vi "Test Decimation.vi"() -> ()   [LabVIEW 2019]
uses:
  <vilib>/Analysis/baseanly.llb/Mean (DBL).vi
  <vilib>/Utility/error.llb/Clear Errors.vi
  <vilib>/Analysis/2dsp.llb/Decimate (single shot).vi
  <vilib>/Analysis/2dsp.llb/Decimate (single shot, DBL).vi
  src/DSP/Factorize Integer.vi
  <vilib>/measure/NI_MABase.lvlib
  src/DSP/DSP.lvclass
  <vilib>/Analysis/NI_AALBase.lvlib
panel:
  out "Decimation Factor":i32
  out "Waveform Graph":waveform(dbl)[](graph)
  out "XY Graph 2":cluster{i32[], dbl[]}[](graph)
  out "elapsed":dbl
  out "Method (0/1/2)":i32
  out "Decimating":i32
  out "Fs":dbl
  out "XY Graph":cluster{"Fs":dbl[], dbl[]}[](graph)
  out "Average Time\n(Decimate, Multistage, Array)":dbl[](array[numeric]) format="%#_6p"
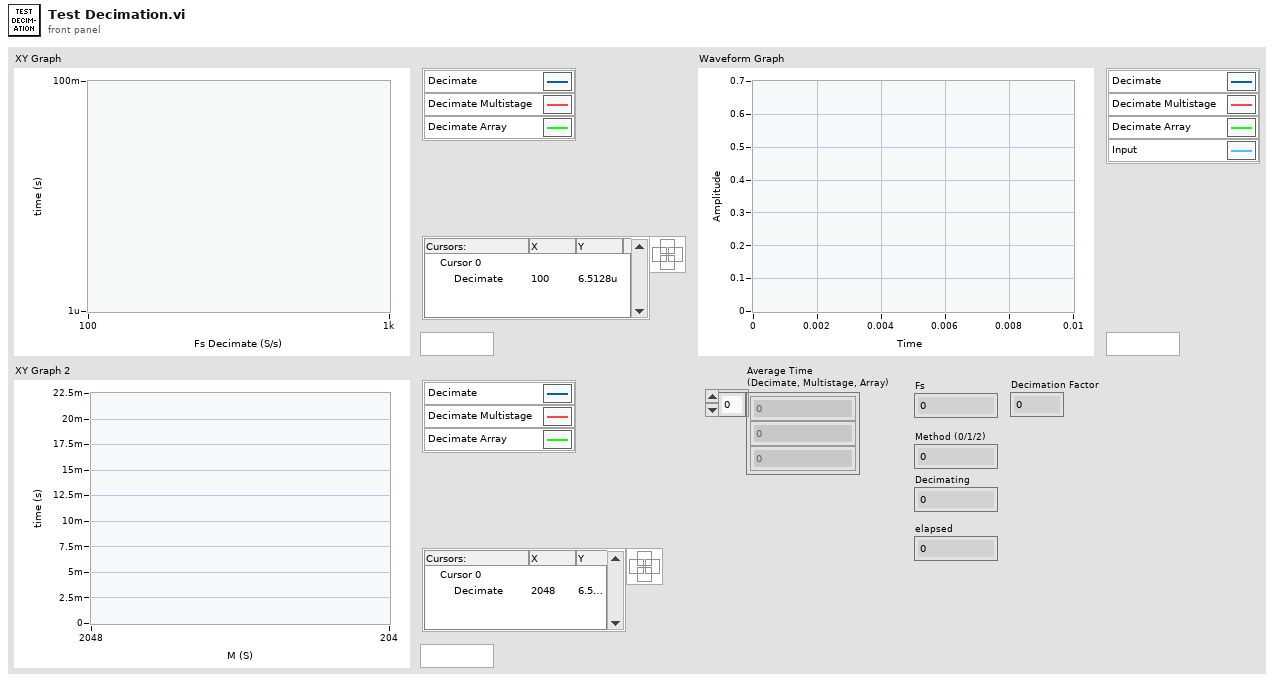
[diagram p1: front panel]
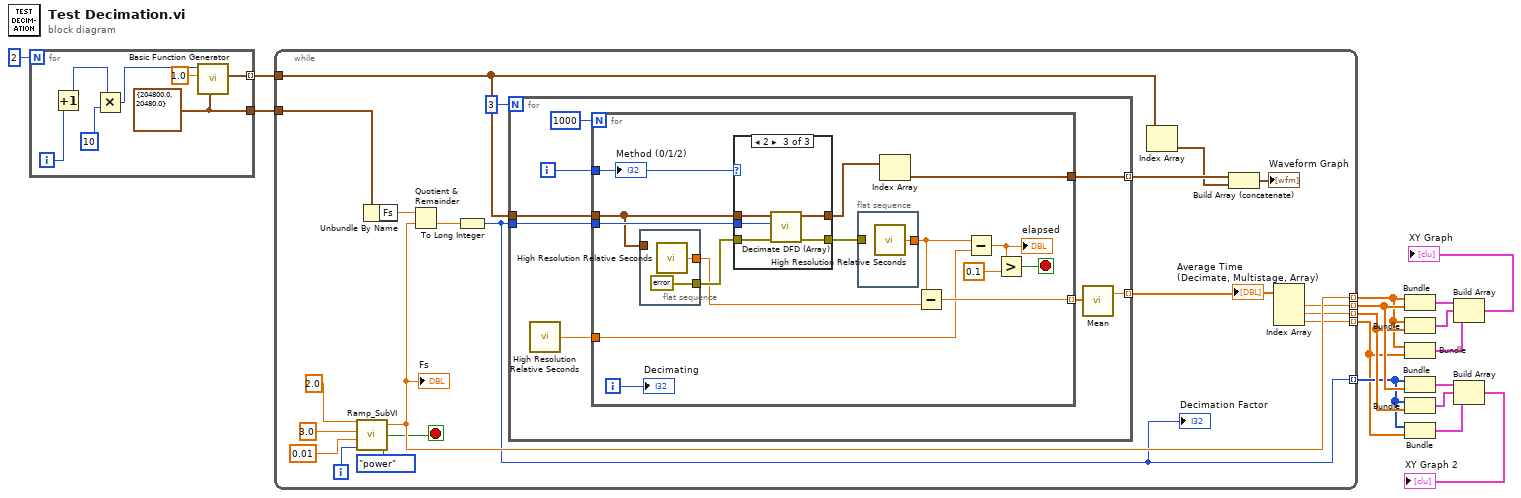
[diagram p0: block diagram]
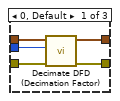
[diagram p2: hidden frame]
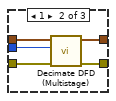
[diagram p3: hidden frame]
diagram:
  n1 = for {
    N: 2 -> [_]
    tunnel: [w23] -> w1 mode=indexing
    tunnel: [w21] -> w15
    i -> [w22]
    w21 = cluster{"Fs":dbl, "#s":dbl} {"Fs"=204800.0, "#s"=20480.0} ("sampling info")
    n2 = Increment(x=w22) -> (x+1=w18:i32)
    n3 = Multiply(x=w18, y=10) -> (x*y=w17:i32)
    n4 = call <vilib>:"Basic Function Generator.vi"("sampling info"=w21, "amplitude"=1.0, "frequency"=w17) -> ("signal out"=w23:waveform(dbl))  [unwired: 6 in, 2 out]
  }
  n5 = while {
    tunnel: w1 -> [w24]
    tunnel: w15 -> [w25]
    tunnel: [w40] -> w5 mode=indexing
    tunnel: [w34] -> w11 mode=indexing
    tunnel: [w26] -> w6 mode=indexing
    tunnel: [w33] -> w10 mode=indexing
    tunnel: [w31] -> w4 mode=indexing
    i -> [w39]
    stop <- w27 stop-if-true
    n6 = call <userlib>:"Ramp_SubVI.vi"("Enum"=enum16{"linear", "power"}."power", "index"=w39, "step"=0.01, "end"=3.0, "start"=2.0) -> ("Stop?"=w27:bool, "Numeric"=w40:dbl)
    "Fs" <- w40
    n7 = Unbundle By Name(w25) -> ("Fs"=w42:dbl)
    n8 = Quotient & Remainder(x=w42, y=w40) -> (floor(x/y)=w32:dbl)  [unwired: 1 out]
    n9 = To Long Integer(number=w32) -> (32bit integer=w26:i32)
    "Decimation Factor" <- w26
    n10 = for {
      N: 3 -> [_]
      tunnel: w24 -> [w48]
      tunnel: [w46] -> w41 mode=indexing
      tunnel: w26 -> [w49]
      tunnel: [w44] -> w29 mode=indexing
      i -> [w50]
      n11 = call <vilib>:"High Resolution Relative Seconds.vi"() -> ("relative seconds"=w45:dbl)
      n12 = for {
        N: 1000 -> [_]
        tunnel: w50 -> [w66]
        tunnel: w49 -> [w65]
        tunnel: w48 -> [w52]
        tunnel: [w57] -> w47 mode=indexing
        tunnel: w45 -> [w55]
        tunnel: [w53] -> w44
        i -> [w61]
        stop <- w63 stop-if-true
        n13 = flat-sequence {
          tunnel: [w68] -> w58
          tunnel: w52 -> [_]
          tunnel: [errorcluster {"status"=FALSE, "code"=0, "source"=""} ("error in (no error)")] -> w59
          frame #0 {
            n14 = call <vilib>:"High Resolution Relative Seconds.vi"() -> ("relative seconds"=w68:dbl)
          }
        }
        n15 = case shown="2" w66 {
          tunnel: w52 -> [w74 w79 w84]
          tunnel: [w73 w78 w81] -> w60
          tunnel: w65 -> [w72 w77 w82]
          tunnel: w59 -> [w71 w76 w83]
          tunnel: [w70 w75 w80] -> w54
          frame 0, Default {
            n16 = call "Decimate DFD (Decimation Factor).vi"("error in (no error)"=w71, "Decimation Factor"=w72, "Waveforms in"=w74) -> ("error out"=w73:errorcluster, "waveforms out"=w70:waveform(dbl)[])  [unwired: 7 in]
          }
          frame 1 {
            n17 = call "Decimate DFD (Multistage).vi"("error in (no error)"=w76, "Decimation Factor"=w77, "Waveforms in"=w79) -> ("error out"=w78:errorcluster, "waveforms out"=w75:waveform(dbl)[])  [unwired: 7 in]
          }
          frame 2 {
            n18 = call "Decimate DFD (Array).vi"("error in (no error)"=w83, "Decimation Factor"=w82, "Waveforms in"=w84) -> ("error out"=w81:errorcluster, "waveforms out"=w80:waveform(dbl)[])  [unwired: 7 in]
          }
        }
        n19 = flat-sequence {
          tunnel: [w69] -> w56
          tunnel: w60 -> [_]
          frame #0 {
            n20 = call <vilib>:"High Resolution Relative Seconds.vi"() -> ("relative seconds"=w69:dbl)
          }
        }
        n21 = Index Array(array=w54) -> (element=w53:waveform(dbl))  [unwired: 1 in]
        n22 = Subtract(x=w56, y=w58) -> (x-y=w57:dbl)
        n23 = Subtract(x=w56, y=w55) -> (x-y=w64:dbl)
        "elapsed" <- w64
        n24 = Greater?(x=w64, y=0.1) -> (0:w63:bool)
        "Decimating" <- w61
        "Method (0/1/2)" <- w66
      }
      n25 = call-poly <vilib>:"Mean.vi"("X"=w47) -> ("mean"=w46:dbl)  [unwired: 1 out]
    }
    "Average Time\n(Decimate, Multistage, Array)" <- w41
    n26 = Index Array(array=w24) -> (element=w28:waveform(dbl))  [unwired: 1 in]
    n27 = Build Array (concatenate)(w29, w28) -> (→"Waveform Graph":waveform(dbl)[])
    n28 = Index Array(array=w41) -> (element #1=w34:dbl, element #2=w33:dbl, element #3=w31:dbl)  [unwired: 3 in]
  }
  n29 = Bundle(w5, w11) -> (w8:cluster{dbl[], dbl[]})  [unwired: 1 in]
  n30 = Bundle(w5, w10) -> (w9:cluster{dbl[], dbl[]})  [unwired: 1 in]
  n31 = Bundle(w5, w4) -> (w3:cluster{dbl[], dbl[]})  [unwired: 1 in]
  n32 = Bundle(w6, w11) -> (w13:cluster{i32[], dbl[]})  [unwired: 1 in]
  n33 = Bundle(w6, w10) -> (w7:cluster{i32[], dbl[]})  [unwired: 1 in]
  n34 = Bundle(w6, w4) -> (w2:cluster{i32[], dbl[]})  [unwired: 1 in]
  n35 = Build Array(w8, w9, w3) -> (→"XY Graph":cluster{dbl[], dbl[]}[])
  n36 = Build Array(w13, w7, w2) -> (→"XY Graph 2":cluster{i32[], dbl[]}[])
